vi "EP_SP.vi"(8 "error in":errorcluster, 10 "new_position":i32, 11 "VISA in":refnum<visa-resource-name>) -> (0 "error out":errorcluster, 3 "VISA out":refnum<visa-resource-name>)   [LabVIEW 2019]
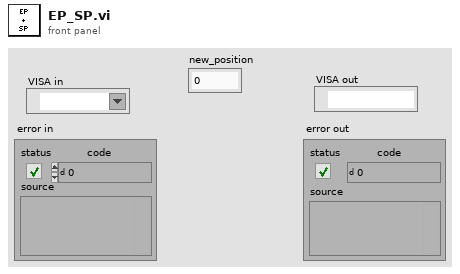
[diagram p1: front panel]
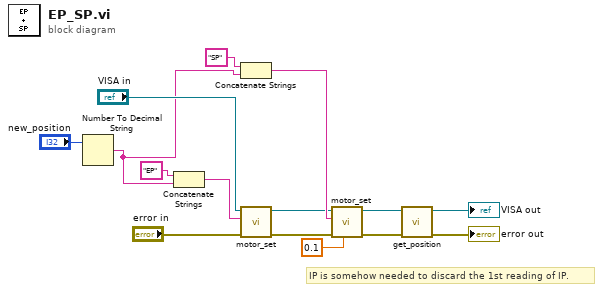
[diagram p0: block diagram]
diagram:
  # "IP is somehow needed to discard the 1st reading of IP."
  n1 = Number To Decimal String(number="new_position") -> (decimal integer string=w7:string)  [unwired: 1 in]
  n2 = Concatenate Strings("EP", w7) -> (w15:string)
  n3 = Concatenate Strings("SP", w7) -> (w9:string)
  n4 = call "motor_set.vi"("error in"="error in", "command"=w15, "VISA in"="VISA in") -> ("error out"=w6:errorcluster, "VISA out"=w8:refnum<visa-resource-name>)  [unwired: 7 in]
  n5 = call "motor_set.vi"("delay  (sec)"=0.1, "error in"=w6, "command"=w9, "VISA in"=w8) -> ("error out"=w4:errorcluster, "VISA out"=w2:refnum<visa-resource-name>)  [unwired: 6 in]
  n6 = call "get_position.vi"("error in"=w4, "VISA"=w2) -> ("error out"=→"error out":errorcluster, "VISA out"=→"VISA out":refnum<visa-resource-name>)  [unwired: 6 in, 2 out]
